vi "TESTGU.vi"() -> ()   [LabVIEW 2013]
uses:
  Device Drivers/DG645/subVIs/channels_TypDef.ctl
  DelayControl2.ctl
  DelaYTypDef.ctl
panel:
  in  "output cluster 2":T1 {"Delay" format="%+.12f"}
  in  "Numeric 15":T3 format="%+.12f"
  in  "Numeric 14":T3 format="%+.12f"
  in  "Numeric 13":T3 format="%+.12f"
  in  "Numeric 12":T3 format="%+.12f"
  in  "Linked.Ch A":T2
  # "T0"
  # "T1"
  # "A"
  # "B"
  # "C"
  # "D"
  # "E"
  # "F"
  # "G"
  # "H"
  # "+"
  # "="
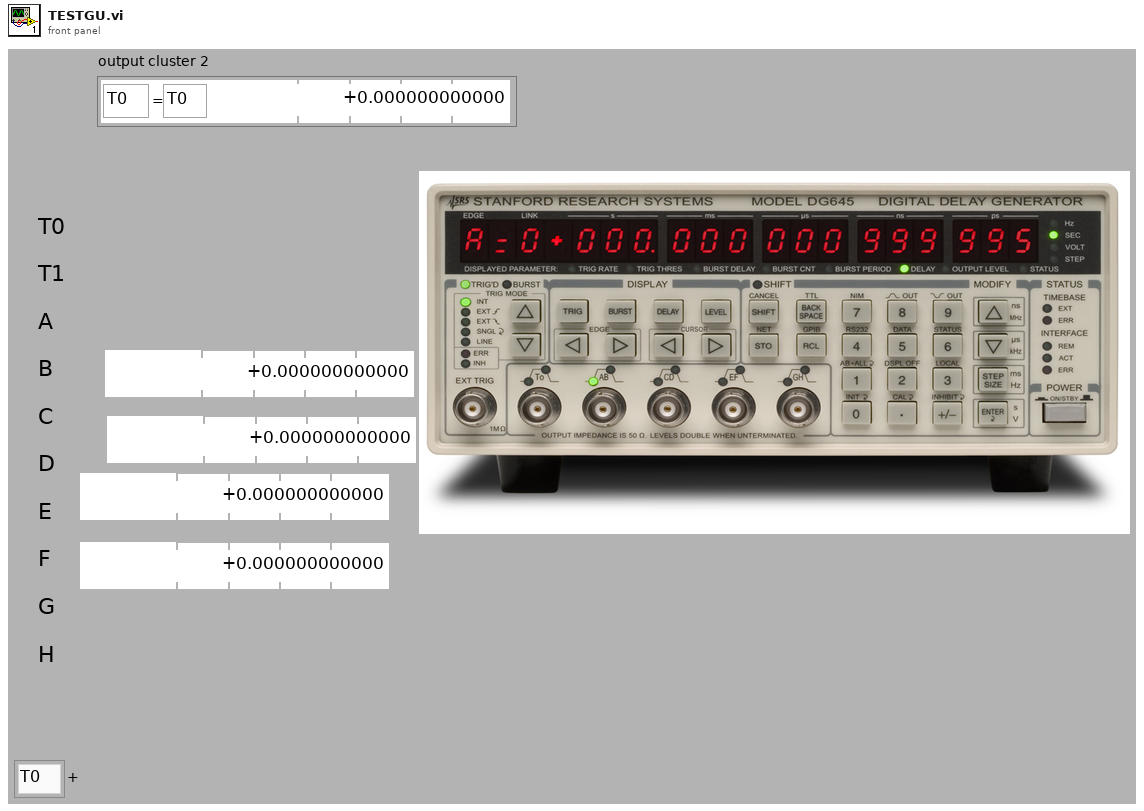
[diagram p1: front panel]
types:
  T1 = typedef "DelaYTypDef.ctl" = cluster{"Ch":T2, "Linked.":T2, "Delay":T3}
  T2 = typedef "channels_TypDef.ctl" = enum16{"T0", "T1", "A", "B", "C", "D", "E", "F", "G", "H"}
  T3 = typedef "DelayControl2.ctl" = dbl
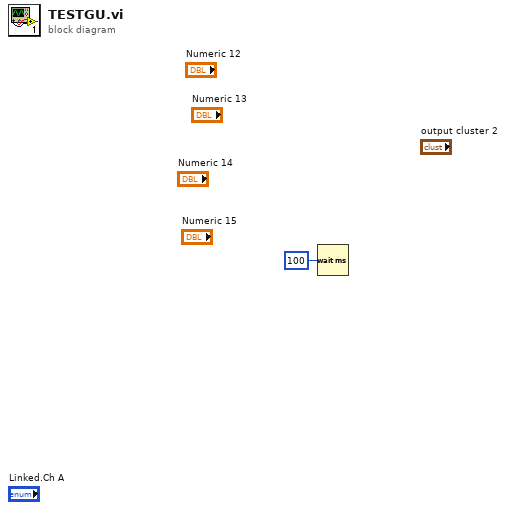
[diagram p0: block diagram]
diagram:
  n1 = Wait (ms)(milliseconds to wait=u32 100) -> ()  [unwired: 1 out]
